vi "getRuns.vi"(8 "error in (no error)":errorcluster, 11 "xwpfParagraph in":refnum<class "xwpfParagraph.lvclass">) -> (0 "error out":errorcluster, 3 "xwpfParagraph out":refnum<class "xwpfParagraph.lvclass">)   [LabVIEW 2017, in "Word_Specific.lvlib" / "xwpfParagraph.lvclass"]
uses:
  xwpfParagraph.lvclass
  xwpfParagraph.lvclass/xwpfParagraph.ctl
  C:/Users/Neo/Desktop/Dev_Tools_BR/LabVIEW_NPOI/lib/NPOI 2.1.1/NPOI.OOXML.dll
  lib/NPOI 2.1.1/NPOI.OOXML.dll
  xwpfRun/xwpfRun.lvclass
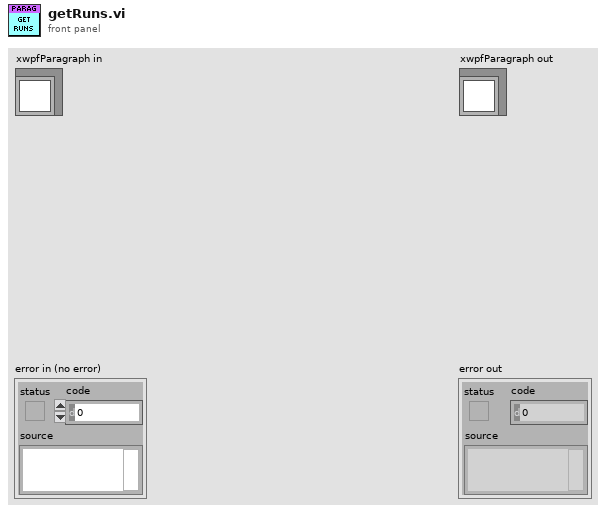
[diagram p1: front panel]
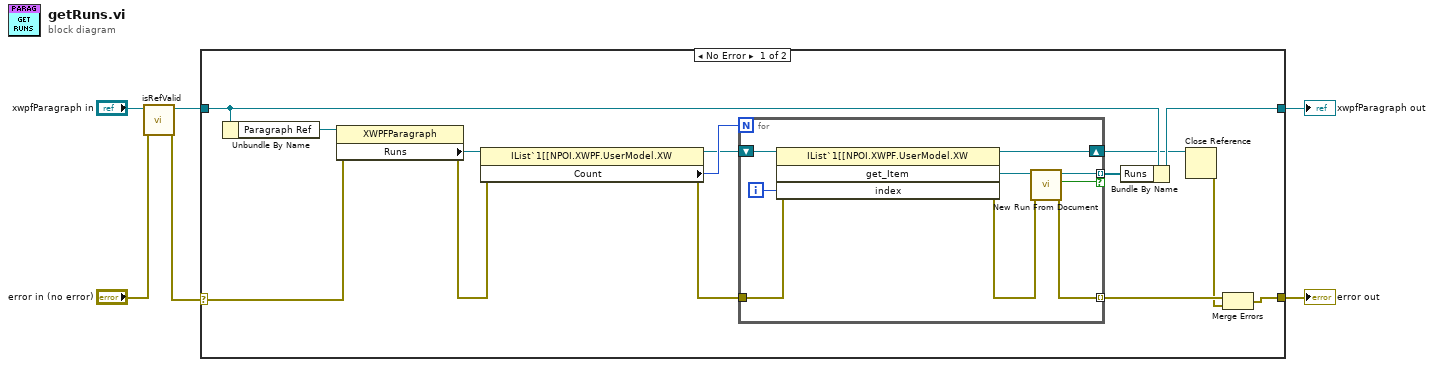
[diagram p0: block diagram]
diagram:
  n1 = call-dynamic "isRefValid.vi"("error in (no error)"="error in (no error)", "xwpfParagraph in"="xwpfParagraph in") -> ("error out"=w1:errorcluster, "xwpfParagraph out"=w3:refnum<class "xwpfParagraph.lvclass">)  [unwired: 8 in]
  n2 = case shown="No Error" w1 {
    selector: w1 -> [w19 w31]
    tunnel: [w13 w31] -> w6
    tunnel: [w11 w30] -> w4
    tunnel: w3 -> [w12 w30]
    frame No Error {
      n3 = Unbundle By Name(w12) -> ("Paragraph Ref"=w20:refnum<k24>)
      n4 = property class="XWPFParagraph"(reference=w20, error in=w19) -> (error out=w16:errorcluster, "Runs"=w18:refnum<k24>)  [unwired: 1 out]
      n5 = property class="IList`1[[NPOI.XWPF.UserModel.XW"(reference=w18, error in=w16) -> (reference out=w7:refnum<k24>, error out=w15:errorcluster, "Count"=w17:i32)
      n6 = for {
        N: w17 -> [_]
        shift-right: [w23] -> w9
        shift-left: w7 -> [w29]
        tunnel: w15 -> [w28]
        tunnel: [w27] -> w10 mode=indexing if=w22
        tunnel: [w25] -> w14 mode=indexing
        i -> [w24]
        n7 = invoke class="IList`1[[NPOI.XWPF.UserModel.XW" method="get_Item"(reference=w29, error in=w28, "index"=w24) -> (reference out=w23:refnum<k24>, error out=w26:errorcluster, "get_Item"=w21:refnum<k24>)  [unwired: 1 in, 1 out]
        n8 = call "New Run From Document.vi"("error in (no error)"=w26, "Run Ref"=w21) -> ("error out"=w25:errorcluster, "New Element Found"=w22:bool, "xwpfRun out"=w27:refnum<class "xwpfRun.lvclass">)  [unwired: 7 in]
      }
      n9 = Bundle By Name(cluster=w12, "Runs"=w10) -> (w11:refnum<class "xwpfParagraph.lvclass">)
      n10 = Close Reference(reference=w9) -> (error out=w8:errorcluster)  [unwired: 1 in]
      n11 = Merge Errors(w14, w8) -> (w13:errorcluster)
    }
    frame Error {
    }
  }
  "error out" <- w6
  "xwpfParagraph out" <- w4
